vi "loadImageAndConvert.vi"(7 "image path":path, 8 "error in (no error)":errorcluster, 10 "name or relative path":string) -> (0 "error out":errorcluster, 2 ".NET object":refnum<k24>)   [LabVIEW 2016, in "DataGrid.lvlib" / "DataTable.lvclass"]
uses:
  <userlib>/LabVIEWdotNetDataGrid/source/DataTable/DataTable.lvclass
  System.Drawing
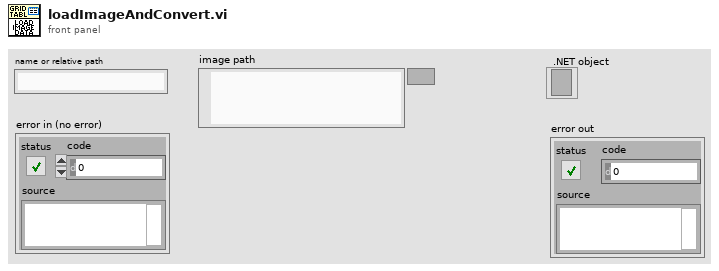
[diagram p1: front panel]
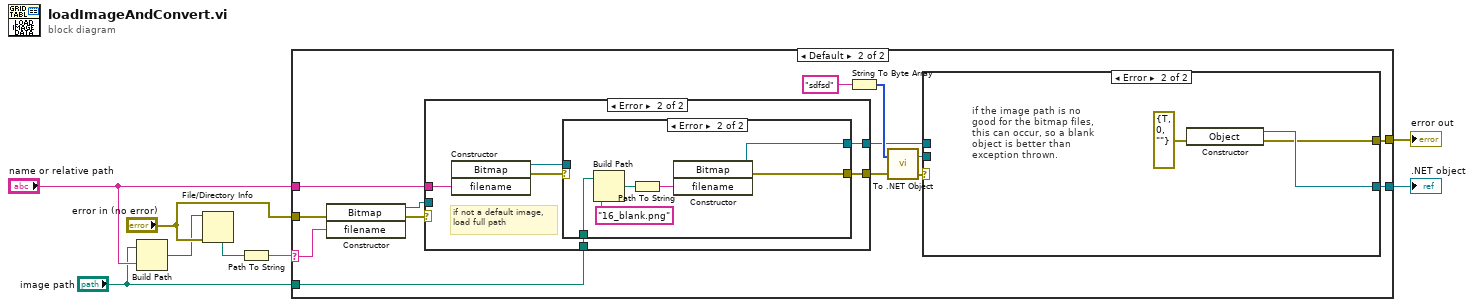
[diagram p0: block diagram]
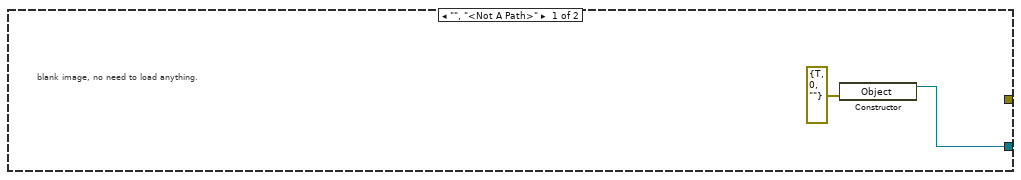
[diagram p2: hidden frame]
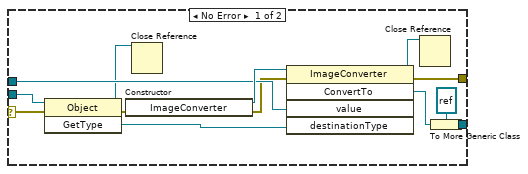
[diagram p3: hidden frame]
diagram:
  n1 = Build Path(base path="image path", name or relative path="name or relative path") -> (appended path=w2:path)
  n2 = File/Directory Info(path=w2, error in="error in (no error)") -> (resolved path=w4:path)  [unwired: 6 out]
  n3 = Path To String(path=w4) -> (string=w5:string)
  n4 = case shown="Default" w5 {
    selector: w5 -> [_ w13]
    tunnel: [w9 w18] -> w8
    tunnel: [_ w17] -> w7
    tunnel: "image path" -> [_ w16]
    tunnel: "name or relative path" -> [_ w14]
    tunnel: "error in (no error)" -> [_ w12]
    frame "", "<Not A Path>" {
      # "blank image, no need to load anything."
      n5 = constructor class="Object"(error in=errorcluster {"status"=TRUE, "code"=0, "source"=""} ("error in (no error)")) -> (reference out=w9:refnum<k24>)  [unwired: 2 in, 2 out]
    }
    frame Default {
      n6 = constructor class="Bitmap"(error in=w12, "filename"=w13) -> (reference out=w24:refnum<k24>, error out=w15:errorcluster)  [unwired: 2 in, 2 out]
      n7 = case shown="Error" w15 {
        tunnel: w14 -> [_ w47]
        tunnel: [w41 w45] -> w21
        tunnel: w24 -> [w41 _]
        tunnel: [_ w44] -> w19
        tunnel: w16 -> [_ w42]
        frame No Error {
          # "Used when a filename is given."
        }
        frame Error {
          # "if not a default image,\nload full path"
          n8 = constructor class="Bitmap"("filename"=w47) -> (reference out=w43:refnum<k24>, error out=w46:errorcluster)  [unwired: 3 in, 2 out]
          n9 = case shown="Error" w46 {
            selector: w46 -> [w48 _]
            tunnel: [w49 w55] -> w45
            tunnel: [w48 w54] -> w44
            tunnel: w43 -> [w49 _]
            tunnel: w42 -> [_ w50]
            frame No Error {
            }
            frame Error {
              n10 = Build Path(base path=w50, name or relative path="16_blank.png" ("filename")) -> (appended path=w53:path)
              n11 = Path To String(path=w53) -> (string=w52:string)
              n12 = constructor class="Bitmap"("filename"=w52) -> (reference out=w55:refnum<k24>, error out=w54:errorcluster)  [unwired: 3 in, 2 out]
            }
          }
        }
      }
      n13 = String To Byte Array(string="sdfsd") -> (unsigned byte array=w22:u8[])
      n14 = call <vilib>:"To .NET Object.vi"("error in (no error)"=w19, "anything"=w22) -> ("error out"=w11:errorcluster, ".NET object"=w23:refnum<k24>)
      n15 = case shown="Error" w11 {
        selector: w11 -> [w26 _]
        tunnel: w23 -> [w25 _]
        tunnel: w21 -> [w34 _]
        tunnel: [w28 w39] -> w18
        tunnel: [w27 w38] -> w17
        frame No Error {
          n16 = invoke class="Object" method="GetType"(reference=w25, error in=w26) -> (reference out=w29:refnum<k24>, error out=w32:errorcluster, "GetType"=w36:refnum<k24>)  [unwired: 1 in]
          n17 = constructor class="ImageConverter"(error in=w32) -> (reference out=w35:refnum<k24>, error out=w31:errorcluster)  [unwired: 2 in, 1 out]
          n18 = Close Reference(reference=w29) -> ()  [unwired: 1 in, 1 out]
          n19 = invoke class="ImageConverter" method="ConvertTo"(reference=w35, error in=w31, "value"=w34, "destinationType"=w36) -> (reference out=w30:refnum<k24>, error out=w27:errorcluster, "ConvertTo"=w33:refnum<k24>)  [unwired: 1 in, 2 out]
          n20 = Close Reference(reference=w30) -> ()  [unwired: 1 in, 1 out]
          n21 = To More Generic Class(target class=refnum<k24> refnum (".NET object"), reference=w33) -> (generic class reference=w28:refnum<k24>)
        }
        frame Error {
          # "if the image path is no\ngood for the bitmap files,\nthis can occur, so a blank\nobject is better than\nexception thrown."
          n22 = constructor class="Object"(error in=errorcluster {"status"=TRUE, "code"=0, "source"=""} ("error in (no error)")) -> (reference out=w39:refnum<k24>, error out=w38:errorcluster)  [unwired: 2 in, 1 out]
        }
      }
    }
  }
  ".NET object" <- w8
  "error out" <- w7
